vi "Pass If Equal.vi"(6 "Delta":variant, 7 "Description":string, 8 "error in (no error)":errorcluster, 9 "Actual":variant, 10 "Expected":variant, 11 "LUnit Test Case In":refnum<class "LUnit Test Case.lvclass">) -> (0 "error out":errorcluster, 3 "LUnit Test Case Out":refnum<class "LUnit Test Case.lvclass">)   [LabVIEW 2020, in "LUnit Test Case.lvclass"]
doc: "Generates a pass result for the calling test method if the inputs are equal. For numeric inputs, a tolerance range may be specified using the Delta input. A description may be provided to the result."
uses:
  LUnit Test Case.lvclass
  Result Classes/Assertion Result/Public/TypeDefs/Assertion Type.ctl
  LUnit Test Case.lvclass/LUnit Test Case.ctl
  Result Classes/Assertion Result/Assertion Result.lvclass/Assertion Result.ctl
  Result Classes/Test Case Result/Test Case Result.lvclass/Test Case Result.ctl
  Result Classes/Method Result/Method Result.lvclass/Method Result.ctl
  Private/SubVIs/Add test result.vi
  Result Classes/Assertion Result/Community/Write Passed.vi
  Result Classes/Assertion Result/Community/Write Message.vi
  Result Classes/Assertion Result/Community/Write Description.vi
  Result Classes/Assertion Result/Community/Write Assertion Type.vi
  Result Classes/Test Case Result/Community/Record Assertion Result.vi
  Result Classes/Method Result/Community/Accessors/Aggregate Assertion Results.vi
  Result Classes/Assertion Result/Public/Read Status.vi
  Result Classes/Assertion Result/Public/Read Message.vi
  Result Classes/Assertion Result/Public/Read Description.vi
  Result Classes/Method Result/Private/SubVIs/Merge Status.vi
  Result Classes/Method Result/Private/SubVIs/Concatenate result strings.vi
  <vilib>/Utility/Data Type/Get Type Information.vi
  <vilib>/Utility/LVClass/Get LV Class Name.vi
  Result Classes/Assertion Result/Assertion Result.lvclass
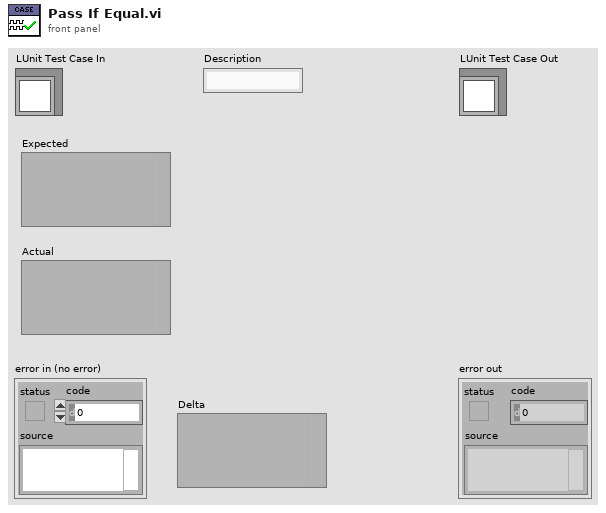
[diagram p1: front panel]
types:
  T1 = typedef "Assertion Result.lvclass/Assertion Type.ctl" = enum16{"None", "Pass", "Fail", "Skip", "Pass if Equal", "Fail if Equal", "Pass if Error", "Fail if Error", "Pass if", "Fail if"}
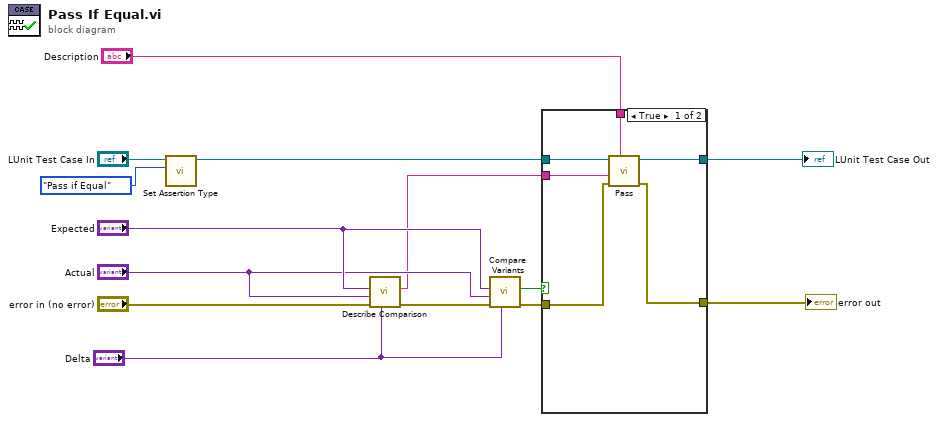
[diagram p0: block diagram]
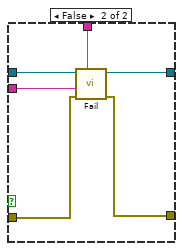
[diagram p2: hidden frame]
diagram:
  n1 = call "Set Assertion Type.vi"("Assertion Type"=Assertion_Type."Pass if Equal", "LUnit Test Case In"="LUnit Test Case In") -> ("LUnit Test Case Out"=w10:refnum<class "LUnit Test Case.lvclass">)  [unwired: 9 in]
  n2 = call "Describe Comparison.vi"("Delta"="Delta", "error in (no error)"="error in (no error)", "Actual"="Actual", "Expected"="Expected") -> ("error out"=w8:errorcluster, "Description"=w2:string)  [unwired: 6 in]
  n3 = call "Compare Variants.vi"("Delta"="Delta", "error in (no error)"=w8, "Actual"="Actual", "Expected"="Expected") -> ("error out"=w6:errorcluster, "Equal?"=w1:bool)  [unwired: 6 in]
  n4 = case shown="True" w1 {
    tunnel: w10 -> [w20 w26]
    tunnel: [w19 w25] -> w13
    tunnel: w6 -> [w18 w24]
    tunnel: "Description" -> [w17 w23]
    tunnel: w2 -> [w16 w22]
    tunnel: [w15 w21] -> w11
    frame True {
      n5 = call "Pass.vi"("Description"=w17, "error in (no error)"=w18, "Message"=w16, "LUnit Test Case In"=w20) -> ("error out"=w15:errorcluster, "LUnit Test Case Out"=w19:refnum<class "LUnit Test Case.lvclass">)  [unwired: 6 in]
    }
    frame False {
      n6 = call "Fail.vi"("Description"=w23, "error in (no error)"=w24, "Message"=w22, "LUnit Test Case In"=w26) -> ("error out"=w21:errorcluster, "LUnit Test Case Out"=w25:refnum<class "LUnit Test Case.lvclass">)  [unwired: 6 in]
    }
  }
  "error out" <- w11
  "LUnit Test Case Out" <- w13
